vi "Trigger.vi"() -> ()   [LabVIEW 2021]
panel:
  out "COUNTDOWN":i32
  in  "stop":bool
  in  "OK Button":bool
  out "Boolean":bool
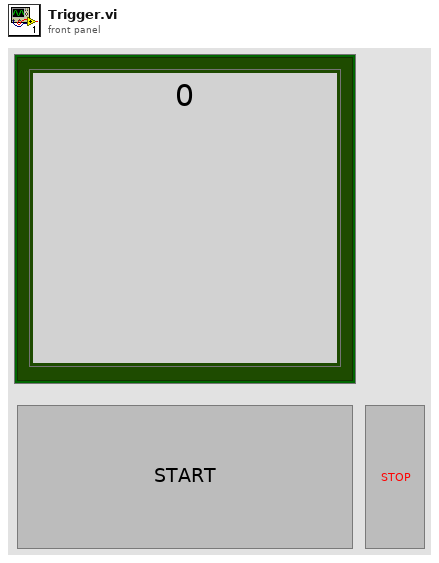
[diagram p1: front panel]
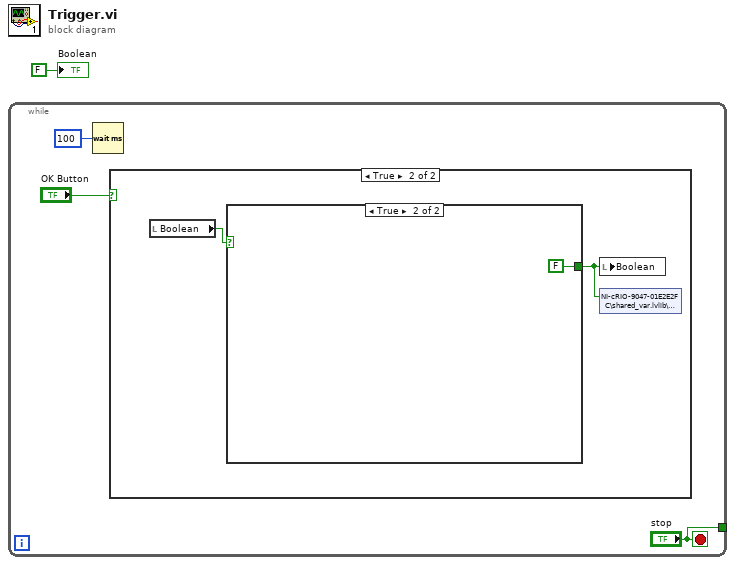
[diagram p0: block diagram]
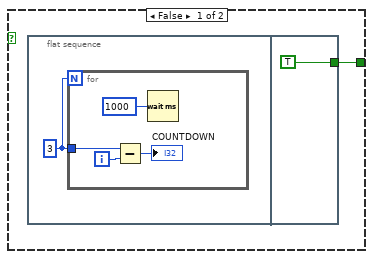
[diagram p3: hidden frame]
diagram:
  n1 = while {
    tunnel: ["stop"] -> _
    stop <- "stop" stop-if-true
    n2 = Wait (ms)(milliseconds to wait=u32 100) -> ()  [unwired: 1 out]
    n3 = case shown="True" "OK Button" {
      frame False {
      }
      frame True {
        n4 = local read "Boolean"() -> (w5:bool)
        n5 = case shown="True" w5 {
          tunnel: [w7 FALSE ("Trigger")] -> w6
          frame False {
            n6 = flat-sequence {
              tunnel: [TRUE ("Trigger")] -> w7
              frame #0 {
                w8 = 3 ("y")
                n7 = for {
                  N: w8 -> [_]
                  tunnel: w8 -> [w10]
                  i -> [w12]
                  n8 = Subtract(x=w10, y=w12) -> (x-y=→"COUNTDOWN":i32)
                  n9 = Wait (ms)(milliseconds to wait=u32 1000) -> ()  [unwired: 1 out]
                }
              }
              frame #1 {
              }
            }
          }
          frame True {
          }
        }
        n10 = local write "Boolean"(w6) -> ()
        n11 = shared-variable "NI-cRIO-9047-01E2E2FC\\shared_var.lvlib\\Trigger"(w6) -> ()  [unwired: 1 in, 1 out]
      }
    }
  }
  "Boolean" <- FALSE ("Boolean")
